vi "Create All Message Queues.vi"(8 "error in (no error)":errorcluster, 11 "Message Queues":T1) -> (0 "error out":errorcluster, 3 "Message Queues out":T1)   [LabVIEW 2017, in "MessageQueue.lvlib"]
doc: "This VI creates and initializes all the message queues for your application. If your application requires more than one message queue, right-click the \"Message Queues\" constant above and select Open Type Def. Add the new Message Queue(s) to the type definition, then initialize them in this VI."
uses:
  MessageQueue.lvlib
  All Message Queues.ctl
  Message Cluster.ctl
  Enqueue Message (Single).vi
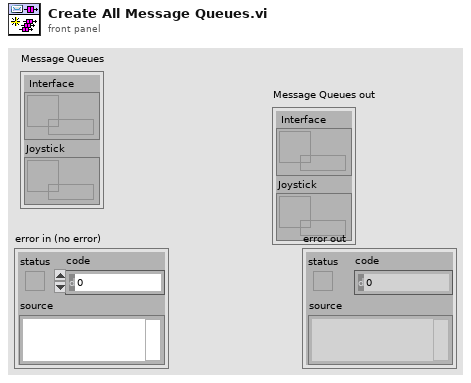
[diagram p1: front panel]
types:
  T1 = typedef "MessageQueue.lvlib/All Message Queues.ctl" = cluster{" Interface":refnum<queue>, "Joystick":refnum<queue>}
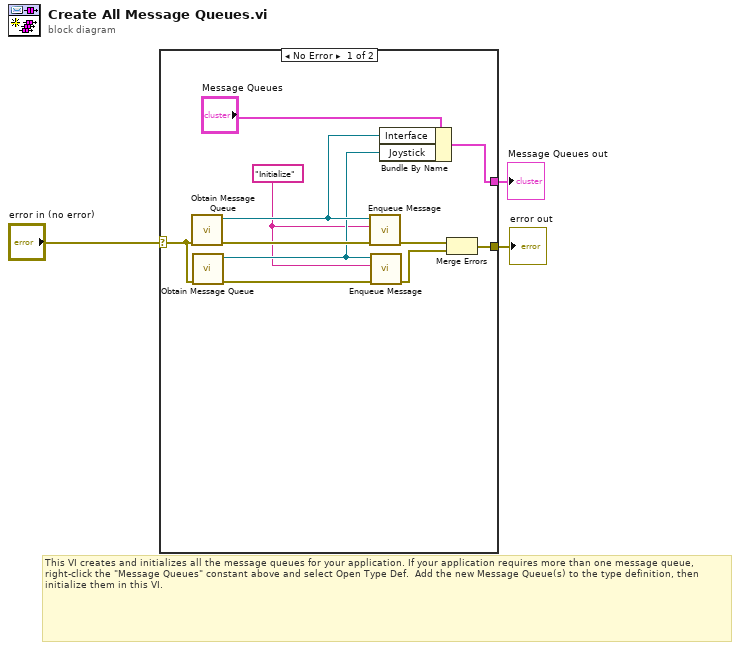
[diagram p0: block diagram]
diagram:
  # "This VI creates and initializes all the message queues for your application. If your application requires more than one message queue, right-click the \"Message Queues\" constant above and select Open Type Def.  Add the new Message Queue(s) to the type definition, then initialize them in this VI."
  n1 = case shown="No Error" "error in (no error)" {
    selector: "error in (no error)" -> [w4 w15]
    tunnel: [w11 w15] -> w3
    tunnel: [w13 _] -> w2
    frame No Error {
      w7 = "Initialize" ("Message")
      n2 = call "Obtain Message Queue.vi"("error in (no error)"=w4) -> ("error out"=w12:errorcluster, "Message Queue"=w9:refnum<queue>)  [unwired: 9 in]
      n3 = call "Obtain Message Queue.vi"("error in (no error)"=w4) -> ("error out"=w10:errorcluster, "Message Queue"=w8:refnum<queue>)  [unwired: 9 in]
      n4 = call-poly "Enqueue Message.vi"("error in (no error)"=w12, "Message"=w7, "Message Queue"=w9) -> ("error out"=w6:errorcluster)  [unwired: 7 in, 1 out]
      n5 = call-poly "Enqueue Message.vi"("error in (no error)"=w10, "Message"=w7, "Message Queue"=w8) -> ("error out"=w5:errorcluster)  [unwired: 7 in, 1 out]
      n6 = Bundle By Name(cluster="Message Queues", "Interface"=w9, "Joystick"=w8) -> (w13:T1)
      n7 = Merge Errors(w6, w5) -> (w11:errorcluster)
    }
    frame Error {
    }
  }
  "Message Queues out" <- w2
  "error out" <- w3
